vi "SavedSettingsRemoveDuplication.vi"(11 "Saved Values":map{string, string}(c390)) -> (2 "Saved Values (parents removed)":map{string, string}(c390), 3 "Saved Values (children removed)":map{string, string}(c390))   [LabVIEW 2019]
uses:
  <vilib>/regexp/Match Regular Expression.xnode
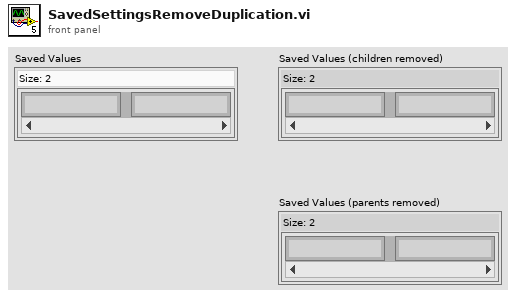
[diagram p1: front panel]
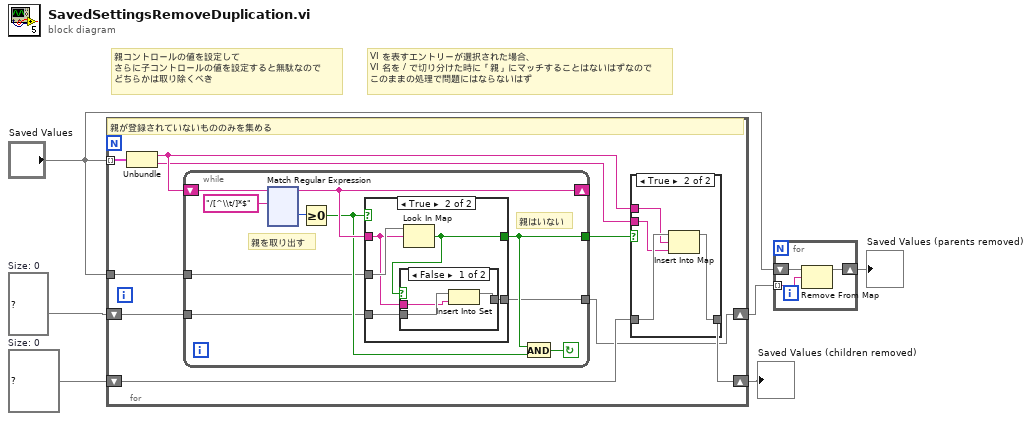
[diagram p0: block diagram]
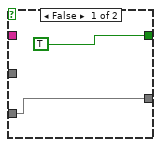
[diagram p3: hidden frame]
diagram:
  w4 = set{string} {}  # Size: 0
  w6 = map{string, string} {}  # Size: 0
  # "VI を表すエントリーが選択された場合、\nVI 名を / で切り分けた時に「親」にマッチすることはないはずなので\nこのままの処理で問題にはならないはず"
  # "親コントロールの値を設定して\nさらに子コントロールの値を設定すると無駄なので\nどちらかは取り除くべき"
  n1 = for {
    tunnel: "Saved Values" -> [w15] mode=indexing
    tunnel: "Saved Values" -> [w14]
    shift-right: [w9] -> w5
    shift-left: w6 -> [w12]
    shift-right: [w7] -> w2
    shift-left: w4 -> [w8]
    # "親が登録されていないもののみを集める"
    n2 = Unbundle(w15) -> (w11:string, w10:string)
    n3 = while {
      shift-right: [w27] -> _
      shift-left: w11 -> [w30]
      tunnel: [w23] -> w13
      tunnel: w14 -> [w24]
      tunnel: w8 -> [w22]
      tunnel: [w21] -> w7
      stop <- w25 continue-if-true
      # "親はいない"
      # "親を取り出す"
      n4 = xnode "Match Regular Expression"("input string"=w30, "regular expression"="/[^\\t/]*$") -> ("before match"=w27:string, "offset past match"=w28:i32)  [unwired: 4 in, 3 out]
      n5 = Greater Or Equal To 0?(x=w28) -> (x >= 0?=w26:bool)
      n6 = case shown="True" w26 {
        tunnel: w27 -> [_ w34]
        tunnel: [TRUE ("key not found?") w36] -> w23
        tunnel: w24 -> [_ w37]
        tunnel: w22 -> [w31 w35]
        tunnel: [w31 w33] -> w21
        frame False {
        }
        frame True {
          n7 = Look In Map(map=w37, key=w34) -> (key not found?=w36:bool)  [unwired: 1 in, 1 out]
          n8 = case shown="False" w36 {
            tunnel: w35 -> [w40 w41]
            tunnel: w34 -> [w39 _]
            tunnel: [w38 w41] -> w33
            frame False {
              n9 = Insert Into Set(10:w39, 11:w40) -> (3:w38:set{string})  [unwired: 1 out]
            }
            frame True {
            }
          }
        }
      }
      n10 = And(x=w23, y=w26) -> (x .and. y?=w25:bool)
    }
    n11 = case shown="True" w13 {
      tunnel: w12 -> [w16 w20]
      tunnel: w11 -> [_ w19]
      tunnel: w10 -> [_ w18]
      tunnel: [w16 w17] -> w9
      frame False {
      }
      frame True {
        n12 = Insert Into Map(map in=w20, key=w19, value=w18) -> (map out=w17:map{string, string})  [unwired: 2 out]
      }
    }
  }
  "Saved Values (children removed)" <- w5
  n13 = for {
    shift-right: [w159] -> w1
    shift-left: "Saved Values" -> [w161]
    tunnel: w2 -> [w160] mode=indexing
    n14 = Remove From Map(10:w160, 11:w161) -> (3:w159:map{string, string})  [unwired: 2 out]
  }
  "Saved Values (parents removed)" <- w1
